vi "FlatToRichveristand_Reponse.vi"(5 "OutputClusterType":T1, 11 "InputCluster":T2) -> (3 "OutputCluster":T1)   [LabVIEW 2020, in "VeriStandgrpc_client.lvlib"]
uses:
  VeriStandgrpc_client.lvlib
  veristand_Reponse_Flat.ctl
  veristand_Reponse.ctl
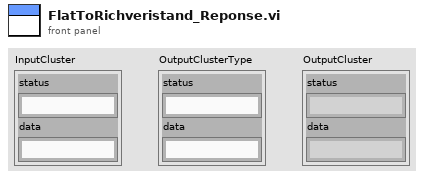
[diagram p1: front panel]
types:
  T1 = typedef "VeriStandgrpc_client.lvlib/veristand_Reponse.ctl" = cluster{"status":string, "data":string}
  T2 = typedef "VeriStandgrpc_client.lvlib/veristand_Reponse_Flat.ctl" = cluster{"status":string, "data":string}
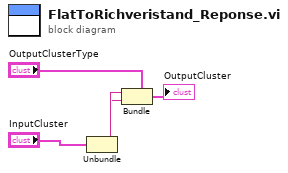
[diagram p0: block diagram]
diagram:
  n1 = Unbundle "Unbundle"("InputCluster") -> ("status"=w2:string, "data"=w1:string)
  n2 = Bundle "Bundle"(cluster="OutputClusterType", "status"=w2, "data"=w1) -> (→"OutputCluster":T1)
